vi "_script_import_template_doc.vi"(11 "md path":path) -> ()   [LabVIEW 2014]
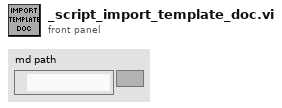
[diagram p1: front panel]
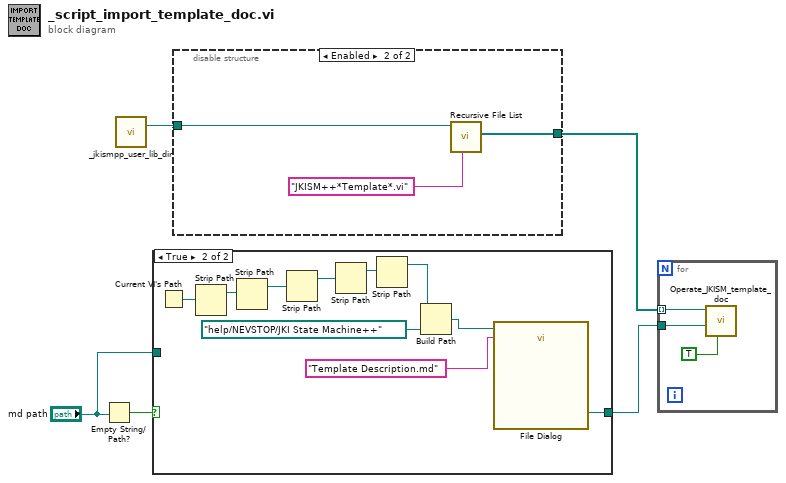
[diagram p0: block diagram]
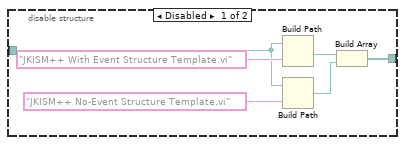
[diagram p3: hidden frame]
diagram:
  n1 = Empty String/Path?(string/path="md path") -> (empty?=w2:bool)
  n2 = call "_jkismpp_user_lib_dir.vi"() -> ("jkismpp_user.lib_dir"=w5:path)  [unwired: 2 in, 1 out]
  n3 = case shown="True" w2 {
    tunnel: [w6 w7] -> w3
    tunnel: "md path" -> [w6 _]
    frame False {
    }
    frame True {
      n4 = Current VI's Path() -> (path=w16:path)
      n5 = Strip Path(path=w16) -> (stripped path=w15:path)  [unwired: 1 out]
      n6 = Strip Path(path=w15) -> (stripped path=w10:path)  [unwired: 1 out]
      n7 = Strip Path(path=w10) -> (stripped path=w13:path)  [unwired: 1 out]
      n8 = Strip Path(path=w13) -> (stripped path=w14:path)  [unwired: 1 out]
      n9 = Strip Path(path=w14) -> (stripped path=w11:path)  [unwired: 1 out]
      n10 = Build Path(base path=w11, name or relative path=path "help/NEVSTOP/JKI State Machine++" ("Path")) -> (appended path=w9:path)
      n11 = call "File Dialog"("start path"=w9, "default name"="Template Description.md") -> ("selected path"=w7:path)  [unwired: 10 in, 3 out]
    }
  }
  n12 = disable-structure shown="Enabled" {
    disable-tunnel: w5 -> [w20 w25]
    disable-tunnel: [w17 w23] -> w4
    frame Disabled {
      n13 = Build Path(base path=w20, name or relative path="JKISM++ With Event Structure Template.vi") -> (appended path=w19:path)
      n14 = Build Path(base path=w20, name or relative path="JKISM++ No-Event Structure Template.vi") -> (appended path=w18:path)
      n15 = Build Array(w19, w18) -> (w17:path[])
    }
    frame Enabled {
      n16 = call <vilib>:"Recursive File List.vi"("pattern"="JKISM++*Template*.vi" ("name or relative path"), "Folder Path"=w25) -> ("All Files in Dir"=w23:path[])  [unwired: 5 in, 4 out]
    }
  }
  n17 = for {
    tunnel: w4 -> [w28] mode=indexing
    tunnel: w3 -> [w27]
    n18 = call "Operate_JKISM_template_doc.vi"("Save to md(F)/Load to vi(T)"=TRUE, "Path"=w27, "vi path"=w28) -> ()  [unwired: 9 in]
  }
